vi "4 intiger comparator.vi"(6 "Numeric 4":i32, 7 "Numeric 3":i32, 8 "Numeric 2":i32, 9 "Numeric":i32) -> (0 "Numeric 8":i32, 1 "Numeric 7":i32, 2 "Numeric 6":i32, 3 "Numeric 5":i32)   [LabVIEW 2012]
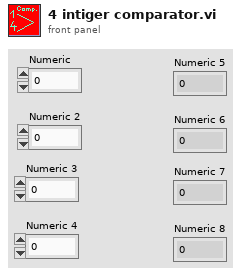
[diagram p1: front panel]
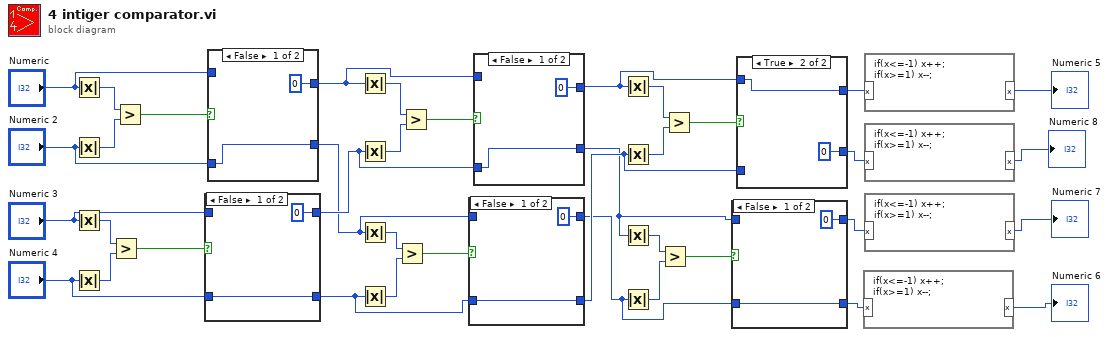
[diagram p0: block diagram]
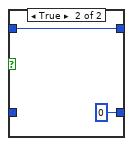
[diagram p2: hidden frame]
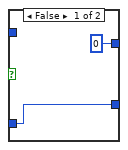
[diagram p3: hidden frame]
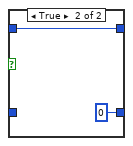
[diagram p4: hidden frame]
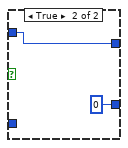
[diagram p5: hidden frame]
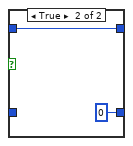
[diagram p6: hidden frame]
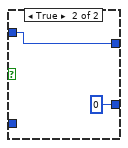
[diagram p7: hidden frame]
diagram:
  n1 = Absolute Value(x="Numeric") -> (abs(x)=w38:i32)
  n2 = Absolute Value(x="Numeric 2") -> (abs(x)=w37:i32)
  n3 = Absolute Value(x="Numeric 3") -> (abs(x)=w36:i32)
  n4 = Absolute Value(x="Numeric 4") -> (abs(x)=w35:i32)
  n5 = Greater?(x=w36, y=w35) -> (0:w31:bool)
  n6 = Greater?(x=w38, y=w37) -> (0:w34:bool)
  n7 = case shown="False" w31 {
    tunnel: "Numeric 3" -> [_ w42]
    tunnel: "Numeric 4" -> [w40 _]
    tunnel: [0 ("Numeric 3") w42] -> w21
    tunnel: [w40 0 ("Numeric 4")] -> w19
    frame False {
    }
    frame True {
    }
  }
  n8 = case shown="False" w34 {
    tunnel: "Numeric" -> [_ w46]
    tunnel: "Numeric 2" -> [w43 _]
    tunnel: [0 ("Numeric") w46] -> w22
    tunnel: [w43 0 ("Numeric 2")] -> w20
    frame False {
    }
    frame True {
    }
  }
  n9 = Absolute Value(x=w22) -> (abs(x)=w28:i32)
  n10 = Absolute Value(x=w21) -> (abs(x)=w27:i32)
  n11 = Absolute Value(x=w20) -> (abs(x)=w26:i32)
  n12 = Absolute Value(x=w19) -> (abs(x)=w25:i32)
  n13 = Greater?(x=w26, y=w25) -> (0:w23:bool)
  n14 = Greater?(x=w28, y=w27) -> (0:w24:bool)
  n15 = case shown="False" w23 {
    tunnel: w20 -> [_ w50]
    tunnel: w19 -> [w48 _]
    tunnel: [0 ("Numeric 3") w50] -> w9
    tunnel: [w48 0 ("Numeric 4")] -> w11
    frame False {
    }
    frame True {
    }
  }
  n16 = case shown="False" w24 {
    tunnel: w22 -> [_ w54]
    tunnel: w21 -> [w51 _]
    tunnel: [0 ("Numeric") w54] -> w12
    tunnel: [w51 0 ("Numeric 2")] -> w10
    frame False {
    }
    frame True {
    }
  }
  n17 = Absolute Value(x=w12) -> (abs(x)=w18:i32)
  n18 = Absolute Value(x=w11) -> (abs(x)=w17:i32)
  n19 = Absolute Value(x=w10) -> (abs(x)=w16:i32)
  n20 = Absolute Value(x=w9) -> (abs(x)=w15:i32)
  n21 = Greater?(x=w16, y=w15) -> (0:w13:bool)
  n22 = Greater?(x=w18, y=w17) -> (0:w14:bool)
  n23 = case shown="False" w13 {
    tunnel: w10 -> [_ w58]
    tunnel: w9 -> [w56 _]
    tunnel: [0 ("Numeric 3") w58] -> w3
    tunnel: [w56 0 ("Numeric 4")] -> w4
    frame False {
    }
    frame True {
    }
  }
  n24 = case shown="True" w14 {
    tunnel: w12 -> [_ w62]
    tunnel: w11 -> [w59 _]
    tunnel: [0 ("Numeric") w62] -> w8
    tunnel: [w59 0 ("Numeric 2")] -> w6
    frame False {
    }
    frame True {
    }
  }
  n25 = formula code="if(x<=-1) x++;\nif(x>=1) x--;"("x"=w4) -> ("x"=→"Numeric 6":i32)
  n26 = formula code="if(x<=-1) x++;\nif(x>=1) x--;"("x"=w8) -> ("x"=→"Numeric 5":i32)
  n27 = formula code="if(x<=-1) x++;\nif(x>=1) x--;"("x"=w6) -> ("x"=→"Numeric 8":i32)
  n28 = formula code="if(x<=-1) x++;\nif(x>=1) x--;"("x"=w3) -> ("x"=→"Numeric 7":i32)
